vi "Example XYGraph Shapes.vi"() -> ()   [LabVIEW 2015]
panel:
  out "XY Graph":cluster{dbl[], dbl[]}[](graph)
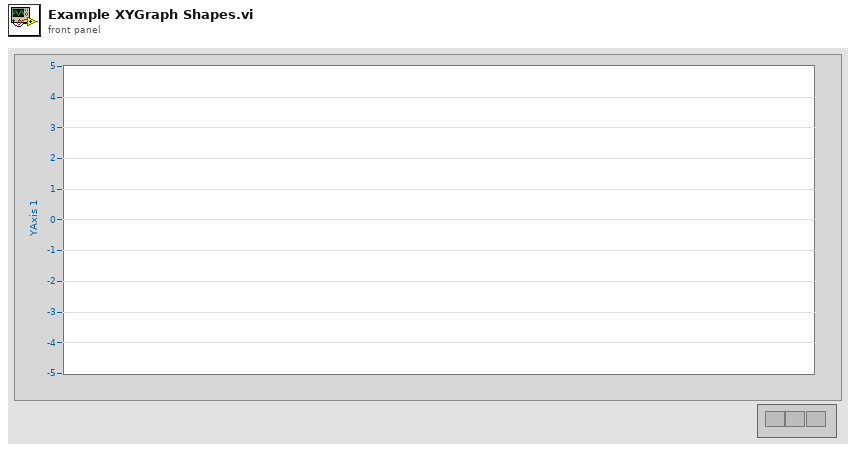
[diagram p1: front panel]
types:
  T1 = typedef "LVPoint32TypeDef.ctl" = cluster{"Horizontal":i32, "Vertical":i32}
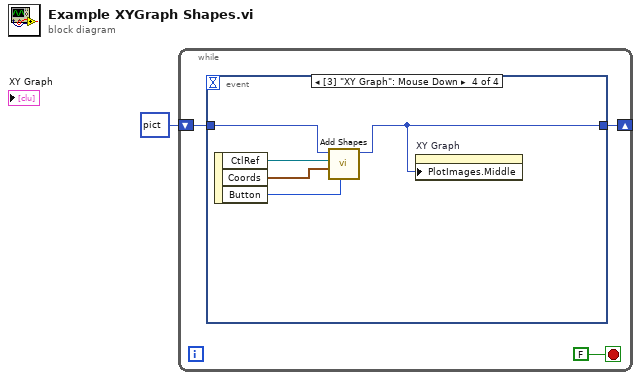
[diagram p0: block diagram]
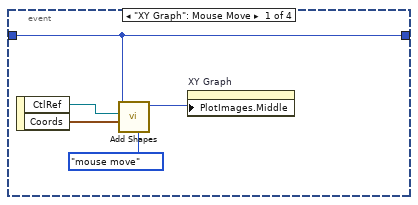
[diagram p2: hidden frame]
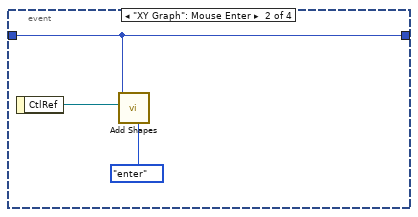
[diagram p3: hidden frame]
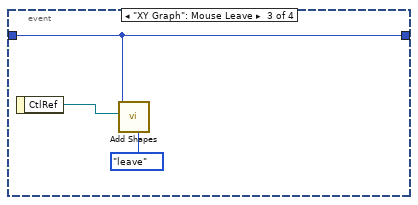
[diagram p4: hidden frame]
diagram:
  n1 = while {
    shift-right: [w2] -> _
    shift-left: picture data[5B] ("output picture") -> [w3]
    stop <- FALSE stop-if-true
    n2 = event shown="[3] \"XY Graph\": Mouse Down" {
      selector: _ -> [_ _ _ _]
      dyn-events: _ -> [_ _ _ _]
      timeout: _ -> [_ _ _ _]
      tunnel: [w6 w11 w14 w16] -> w2
      tunnel: w3 -> [w6 w11 w14 w17]
      event "XY Graph": Mouse Move {
        n3 = event-data() -> ("CtlRef"=w8:refnum<vi>, "Coords"=w9:T1)  [unwired: 1 in]
        n4 = call "Add Shapes.vi"("event"=enum16{"click", "mouse move", "enter", "leave"}."mouse move", "Coords"=w9, "XY Graph"=w8, "input picture"=w6) -> ("output picture"=w7:picture)  [unwired: 6 in, 1 out]
        n5 = property on="XY Graph" class="XYGraph (strict)"("PlotImages.Middle"=w7) -> ()  [unwired: 2 in, 2 out]
      }
      event "XY Graph": Mouse Enter {
        n6 = event-data() -> ("CtlRef"=w12:refnum<vi>)  [unwired: 1 in]
        n7 = call "Add Shapes.vi"("event"=enum16{"click", "mouse move", "enter", "leave"}."enter", "XY Graph"=w12, "input picture"=w11) -> ()  [unwired: 7 in, 2 out]
      }
      event "XY Graph": Mouse Leave {
        n8 = event-data() -> ("CtlRef"=w15:refnum<vi>)  [unwired: 1 in]
        n9 = call "Add Shapes.vi"("event"=enum16{"click", "mouse move", "enter", "leave"}."leave", "XY Graph"=w15, "input picture"=w14) -> ()  [unwired: 7 in, 2 out]
      }
      event "XY Graph": Mouse Down {
        n10 = event-data() -> ("CtlRef"=w20:refnum<vi>, "Coords"=w19:T1, "Button"=w18:u16)  [unwired: 1 in]
        n11 = call "Add Shapes.vi"("Button"=w18, "Coords"=w19, "XY Graph"=w20, "input picture"=w17) -> ("output picture"=w16:picture)  [unwired: 6 in, 1 out]
        n12 = property on="XY Graph" class="XYGraph (strict)"("PlotImages.Middle"=w16) -> ()  [unwired: 2 in, 2 out]
      }
    }
  }
